vi "GeneratePersonnelReport.vi"(8 "Error In":errorcluster) -> (0 "Error Out":errorcluster, 1 "Update":bool, 3 "Array":T1[](array[typedef]))   [LabVIEW 2015]
uses:
  TypeDef/PersonnelReport.ctl
panel:
  in  "Personnel":u16[](array[ring]) items=["Wily", "House", "Jackie", "Florence"]
  in  "Cancel":bool
  in  "Submit":bool
  in  "To":timestamp
  in  "From":timestamp
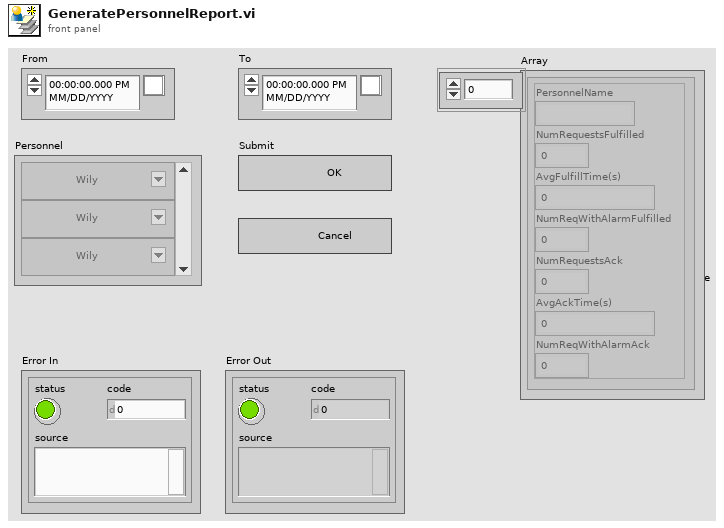
[diagram p1: front panel]
types:
  T1 = typedef "PersonnelReport.ctl" = cluster{"PersonnelName":string, "NumRequestsFulfilled":i32, "AvgFulfillTime(s)":dbl, "NumReqWithAlarmFulfilled":i32, "NumRequestsAck":i32, "AvgAckTime(s)":dbl, "NumReqWithAlarmAck":i32}
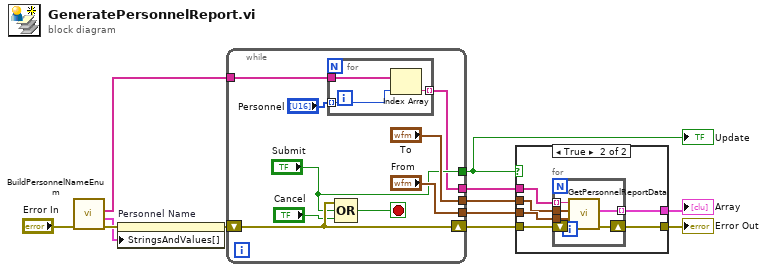
[diagram p0: block diagram]
diagram:
  n1 = call "BuildPersonnelNameEnum.vi"("error in (no error)"="Error In") -> ("error out"=w6:errorcluster, "EnumStringAndVals"=w5:cluster{"String":string, "Value":u16}[], "PUIDs"=w3:string[])  [unwired: 6 in, 2 out]
  n2 = property on="Personnel Name" class="Ring (strict)"(error in=w6, "StringsAndValues[]"=w5) -> (error out=w4:errorcluster)  [unwired: 1 in, 1 out]
  n3 = while {
    shift-right: [w18] -> w11
    shift-left: w4 -> [w18]
    tunnel: ["From"] -> w10
    tunnel: ["To"] -> w9
    tunnel: ["Submit"] -> w8
    tunnel: w3 -> [w15]
    tunnel: [w14] -> w2
    stop <- w19 stop-if-true
    n4 = for {
      tunnel: w15 -> [w24]
      tunnel: [w23] -> w14 mode=indexing
      tunnel: "Personnel" -> [w22] mode=indexing
      n5 = Index Array(array=w24, index=w22) -> (element=w23:string)
    }
    n6 = Compound Arithmetic op=OR(w18, "Submit", "Cancel") -> (w19:bool)
  }
  "Update" <- w8
  n7 = case shown="True" w8 {
    tunnel: [w25 w31] -> w12
    tunnel: w11 -> [w25 w30]
    tunnel: w10 -> [_ w29]
    tunnel: w9 -> [_ w28]
    tunnel: w2 -> [_ w27]
    tunnel: [_ w26] -> w1
    frame False {
    }
    frame True {
      n8 = for {
        tunnel: w29 -> [w35]
        tunnel: w28 -> [w34]
        tunnel: w27 -> [w33] mode=indexing
        tunnel: [w32] -> w26 mode=indexing
        shift-right: [w37] -> w31
        shift-left: w30 -> [w36]
        n9 = call "GetPersonnelReportData.vi"("error in"=w36, "From"=w35, "To"=w34, "PersonnelName"=w33) -> ("error out"=w37:errorcluster, "PersonnelReport"=w32:T1)  [unwired: 6 in]
      }
    }
  }
  "Error Out" <- w12
  "Array" <- w1
